vi "Main-active object.vi"() -> ()   [LabVIEW 2019]
uses:
  active object queue_class/active object queue.lvclass
  Global 1.vi
  adf319f4-8d3a-4dd8-b17c-4e6adddec496.vi
panel:
  out "Attribute1 3":dbl
  out "Status 3":bool
  out "Status 2":bool
  out "Attribute1 2":dbl
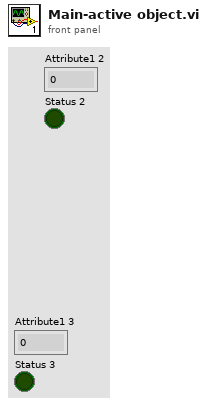
[diagram p1: front panel]
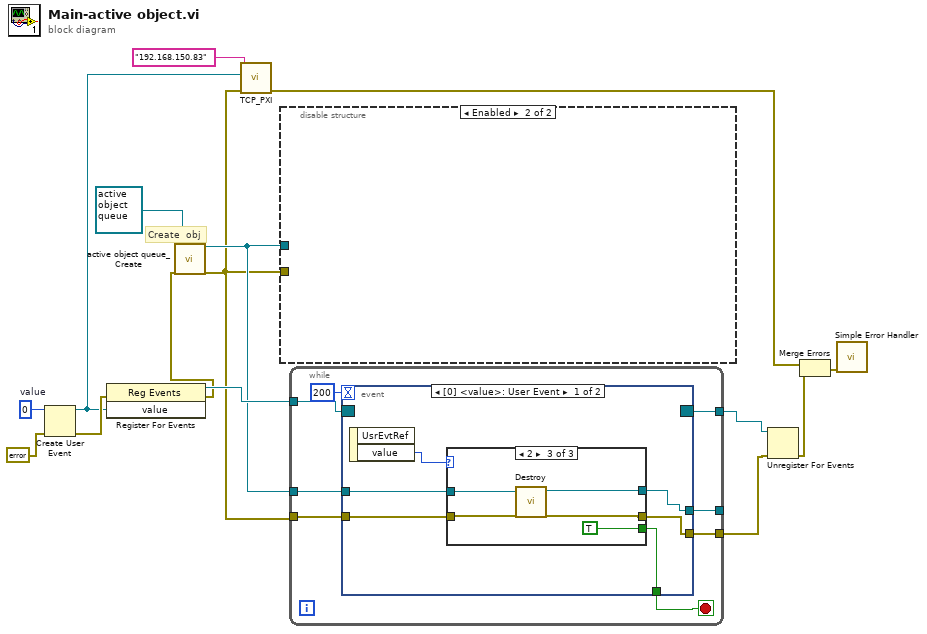
[diagram p0: block diagram]
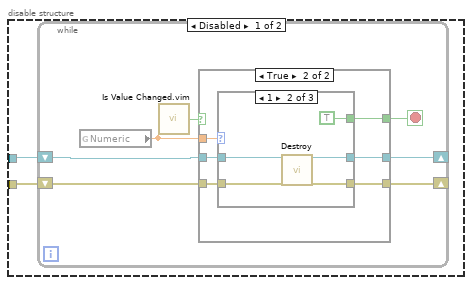
[diagram p2: hidden frame]
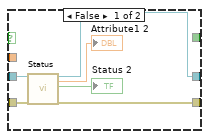
[diagram p3: hidden frame]
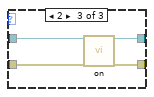
[diagram p5: hidden frame]
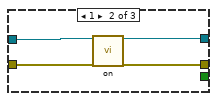
[diagram p7: hidden frame]
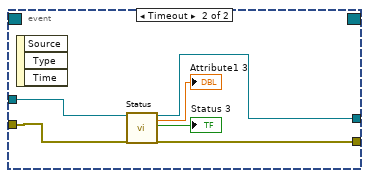
[diagram p8: hidden frame]
diagram:
  w14 = 0  # value
  # "Create  obj"
  n1 = Create User Event(user event datatype=w14, error in=errorcluster {"status"=FALSE, "code"=0, "source"=""} ("error out")) -> (user event=w7:refnum<user-event>, error out=w13:errorcluster)
  n2 = register-events(error in=w13, w7) -> (reference out=w12:refnum<event-registration>, error out=w1:errorcluster)  [unwired: 1 in]
  n3 = call "active object queue_Create.vi"("reference in"=refnum<class "active object queue.lvclass"> refnum ("active object queue"), "error in (no error)"=w1) -> ("reference out"=w11:refnum<class "active object queue.lvclass">, "error out"=w10:errorcluster)  [unwired: 16 in]
  n4 = call "TCP_PXI.vi"("error in (no error) 2"=w10, "user event out"=w7, "Machine"="192.168.150.83") -> ("error out"=w6:errorcluster)  [unwired: 8 in]
  n5 = disable-structure shown="Enabled" {
    disable-tunnel: w11 -> [w17 _]
    disable-tunnel: w10 -> [w16 _]
    frame Disabled {
      n6 = while {
        shift-right: [w21] -> _
        shift-left: w16 -> [w22]
        shift-right: [w20] -> _
        shift-left: w17 -> [w23]
        stop <- w24 stop-if-true
        n7 = global read "Global 1.vi" "Numeric"() -> (w18:dbl)
        n8 = call "Is Value Changed.vim"("value"=w18) -> ("changed or first call?"=w19:bool)
        n9 = case shown="True" w19 {
          tunnel: [_ w36] -> w24
          tunnel: w23 -> [w28 w35]
          tunnel: w22 -> [w27 w34]
          tunnel: [w25 w33] -> w21
          tunnel: [w26 w32] -> w20
          tunnel: w18 -> [_ w31]
          frame False {
            n10 = call-dynamic "Status.vi"("reference in"=w28, "error in (no error)"=w27) -> ("reference out"=w26:refnum<class "active object queue.lvclass">, "Attribute1"=→"Attribute1 2":dbl, "Status"=→"Status 2":bool, "error out"=w25:errorcluster)  [unwired: 14 in]
          }
          frame True {
            n11 = case shown="1" w31 {
              tunnel: w35 -> [w38 w43 w47]
              tunnel: w34 -> [w37 w42 w46]
              tunnel: [w38 w41 w45] -> w32
              tunnel: [w37 w40 w44] -> w33
              tunnel: [_ TRUE _] -> w36
              frame 0, Default {
              }
              frame 1 {
                n12 = call-dynamic "Destroy.vi"("reference in"=w43, "error in (no error)"=w42) -> ("reference out"=w41:refnum<class "active object queue.lvclass">, "error out"=w40:errorcluster)  [unwired: 16 in]
              }
              frame 2 {
                n13 = call "on.vi"("reference in"=w47, "error in (no error)"=w46) -> ("reference out"=w45:refnum<class "active object queue.lvclass">, "error out"=w44:errorcluster)  [unwired: 16 in]
              }
            }
          }
        }
      }
    }
    frame Enabled {
    }
  }
  n14 = while {
    tunnel: w12 -> [w55]
    tunnel: w11 -> [w53]
    tunnel: w10 -> [w52]
    tunnel: [w51] -> _
    tunnel: [w50] -> w8
    tunnel: [w49] -> w9
    stop <- w48 stop-if-true
    n15 = event shown="[0] <value>: User Event" {
      selector: w55 -> [_ _]
      dyn-events: [_ _] -> w49
      timeout: 200 -> [_ _]
      tunnel: w53 -> [w60 w76]
      tunnel: w52 -> [w59 w75]
      tunnel: [w58 w74] -> w51
      tunnel: [w57 w73] -> w50
      tunnel: [w56 _] -> w48
      event User Event {
        n16 = event-data() -> ("value"=w61:i32)  [unwired: 1 in, 1 out]
        n17 = case shown="2" w61 {
          tunnel: [w63 w67 w71] -> w58
          tunnel: [w62 w66 w70] -> w57
          tunnel: w60 -> [w63 w65 w72]
          tunnel: w59 -> [w62 w64 w69]
          tunnel: [_ _ TRUE] -> w56
          frame 0, Default {
          }
          frame 1 {
            n18 = call "on.vi"("reference in"=w65, "error in (no error)"=w64) -> ("reference out"=w67:refnum<class "active object queue.lvclass">, "error out"=w66:errorcluster)  [unwired: 16 in]
          }
          frame 2 {
            n19 = call-dynamic "Destroy.vi"("reference in"=w72, "error in (no error)"=w69) -> ("reference out"=w71:refnum<class "active object queue.lvclass">, "error out"=w70:errorcluster)  [unwired: 16 in]
          }
        }
      }
      event Timeout {
        n20 = event-data() -> ()  [unwired: 1 in, 3 out]
        n21 = call-dynamic "Status.vi"("reference in"=w76, "error in (no error)"=w75) -> ("reference out"=w74:refnum<class "active object queue.lvclass">, "Attribute1"=→"Attribute1 3":dbl, "Status"=→"Status 3":bool, "error out"=w73:errorcluster)  [unwired: 14 in]
      }
    }
  }
  n22 = Unregister For Events(event registration refnum=w9, error in=w8) -> (error out=w5:errorcluster)
  n23 = Merge Errors(w6, w5) -> (w4:errorcluster)
  n24 = call <vilib>:"Simple Error Handler.vi"("error in (no error)"=w4) -> ()  [unwired: 4 in, 5 out]
